vi "230209_Trafficlight_Sync.vi"() -> ()   [LabVIEW 2022 SP3]
panel:
  in  "Standby Off 2":bool
  out "Ampel 2":cluster{"Red":bool, "Orange":bool, "Green":bool}
  out "Ampel":cluster{"Red":bool, "Orange":bool, "Green":bool}
  in  "Ampelzustände Ampel 1":T1(ring)
  in  "Standby Off":bool
  in  "Stop":bool
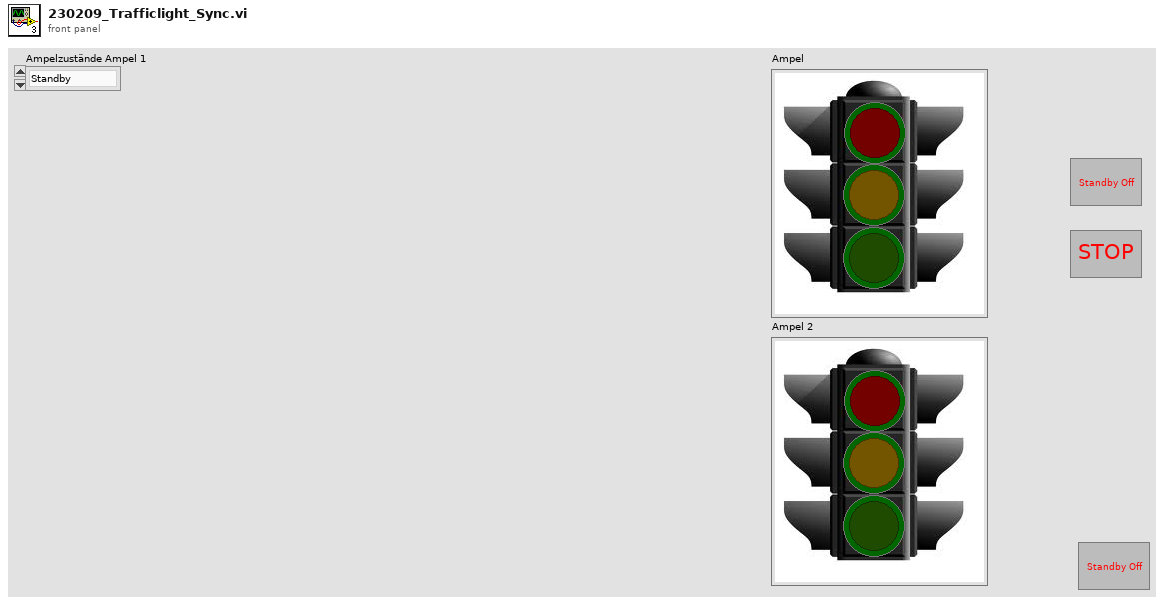
[diagram p1: front panel]
types:
  T1 = enum16{"Standby", "Red", "RedOrange", "Orange", "Green", "GreenBlinking"}
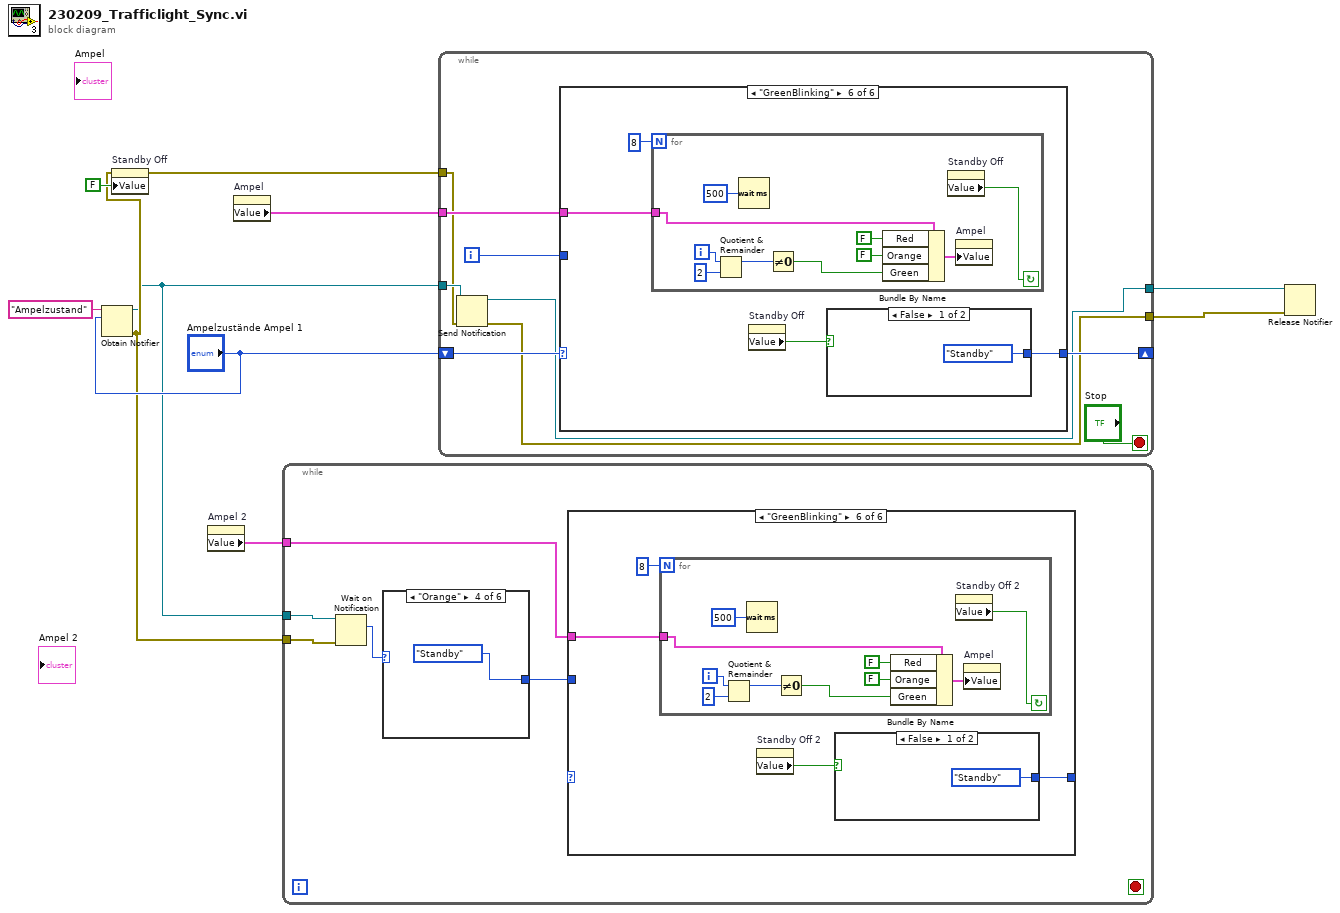
[diagram p0: block diagram]
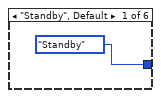
[diagram p2: hidden frame]
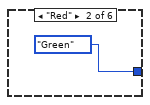
[diagram p3: hidden frame]
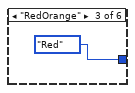
[diagram p4: hidden frame]
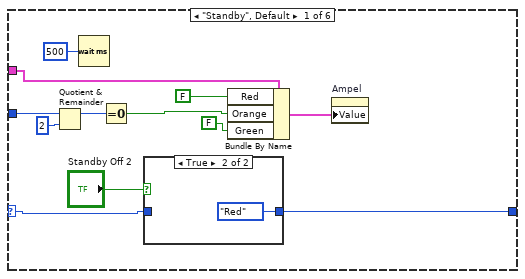
[diagram p7: hidden frame]
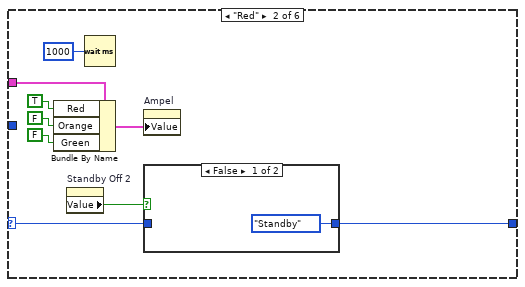
[diagram p9: hidden frame]
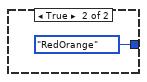
[diagram p10: hidden frame]
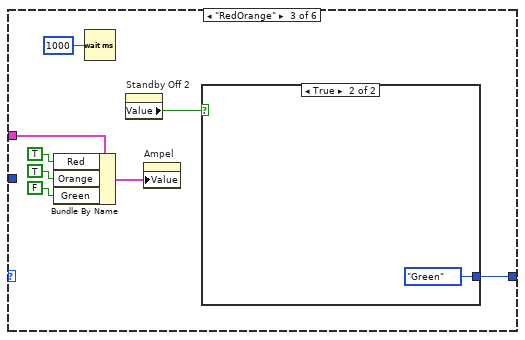
[diagram p11: hidden frame]
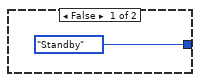
[diagram p12: hidden frame]
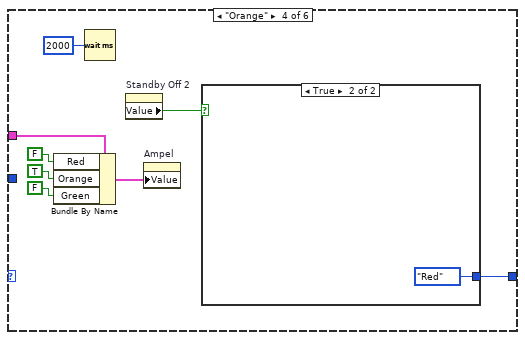
[diagram p13: hidden frame]
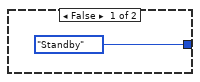
[diagram p14: hidden frame]
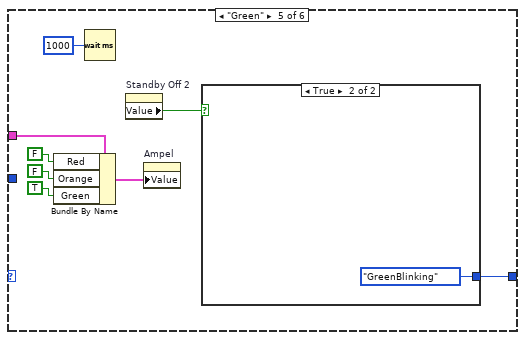
[diagram p15: hidden frame]
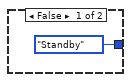
[diagram p16: hidden frame]
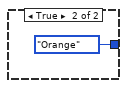
[diagram p17: hidden frame]
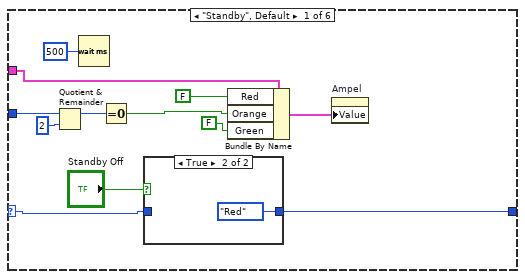
[diagram p18: hidden frame]
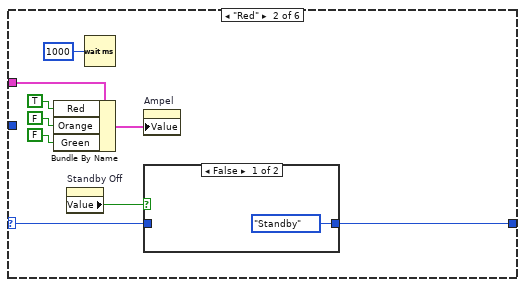
[diagram p20: hidden frame]
diagram:
  n1 = Obtain Notifier(name (unnamed)="Ampelzustand", notification data type="Ampelzustände Ampel 1") -> (notifier out=w2:refnum<notifier>, error out=w3:errorcluster)  [unwired: 2 in, 1 out]
  n2 = property on="Standby Off" class="Bool (strict)"(error in=w3, "Value"=FALSE ("Standby Off")) -> (error out=w8:errorcluster)  [unwired: 1 in, 1 out]
  n3 = property on="Ampel 2" class="Clust (strict)"() -> ("Value"=w1:cluster{"Red":bool, "Orange":bool, "Green":bool})  [unwired: 2 in, 2 out]
  n4 = property on="Ampel" class="Clust (strict)"() -> ("Value"=w10:cluster{"Red":bool, "Orange":bool, "Green":bool})  [unwired: 2 in, 2 out]
  n5 = while {
    tunnel: w3 -> [w15]
    tunnel: w2 -> [w14]
    tunnel: w1 -> [w13]
    stop <- _ stop-if-true
    n6 = Wait on Notification(notifier=w14, error in (no error)=w15) -> (notification=w12:T1)  [unwired: 2 in, 3 out]
    n7 = case shown="\"Orange\"" w12 {
      tunnel: [T1."Standby" ("Enum") T1."Green" ("Enum") T1."Red" ("Enum") T1."Standby" ("Enum") _ _] -> w11
      frame "Standby", Default {
      }
      frame "Red" {
      }
      frame "RedOrange" {
      }
      frame "Orange" {
      }
      frame "Green" {
      }
      frame "GreenBlinking" {
      }
    }
    n8 = case shown="\"GreenBlinking\"" {
      selector: _ -> [w24 w35 _ _ _ _]
      tunnel: w13 -> [w31 w41 w46 w56 w65 w77]
      tunnel: w11 -> [w25 _ _ _ _ _]
      tunnel: [w22 w34 w47 w55 w66 w76] -> _
      frame "Standby", Default {
        n9 = Quotient & Remainder(x=w25, y=2) -> (x-y*floor(x/y)=w27:i32)  [unwired: 1 out]
        n10 = Wait (ms)(milliseconds to wait=u32 500) -> ()  [unwired: 1 out]
        n11 = Equal To 0?(x=w27) -> (x = 0?=w26:bool)
        n12 = case shown="True" "Standby Off 2" {
          tunnel: w24 -> [w32 _]
          tunnel: [w32 T1."Red" ("Enum")] -> w22
          frame False {
          }
          frame True {
          }
        }
        n13 = Bundle By Name(cluster=w31, "Red"=FALSE, "Orange"=w26, "Green"=FALSE) -> (w30:cluster{"Red":bool, "Orange":bool, "Green":bool})
        n14 = property on="Ampel" class="Clust (strict)"("Value"=w30) -> ()  [unwired: 2 in, 2 out]
      }
      frame "Red" {
        n15 = Bundle By Name(cluster=w41, "Red"=TRUE, "Orange"=FALSE, "Green"=FALSE) -> (w42:cluster{"Red":bool, "Orange":bool, "Green":bool})
        n16 = property on="Standby Off 2" class="Bool (strict)"() -> ("Value"=w36:bool)  [unwired: 2 in, 2 out]
        n17 = Wait (ms)(milliseconds to wait=u32 1000) -> ()  [unwired: 1 out]
        n18 = property on="Ampel" class="Clust (strict)"("Value"=w42) -> ()  [unwired: 2 in, 2 out]
        n19 = case shown="False" w36 {
          tunnel: [T1."Standby" ("Enum") T1."RedOrange" ("Enum")] -> w34
          tunnel: w35 -> [_ _]
          frame False {
          }
          frame True {
          }
        }
      }
      frame "RedOrange" {
        n20 = Bundle By Name(cluster=w46, "Red"=TRUE, "Orange"=TRUE, "Green"=FALSE) -> (w45:cluster{"Red":bool, "Orange":bool, "Green":bool})
        n21 = Wait (ms)(milliseconds to wait=u32 1000) -> ()  [unwired: 1 out]
        n22 = property on="Standby Off 2" class="Bool (strict)"() -> ("Value"=w48:bool)  [unwired: 2 in, 2 out]
        n23 = property on="Ampel" class="Clust (strict)"("Value"=w45) -> ()  [unwired: 2 in, 2 out]
        n24 = case shown="True" w48 {
          tunnel: [T1."Standby" ("Enum") T1."Green" ("Enum")] -> w47
          frame False {
          }
          frame True {
          }
        }
      }
      frame "Orange" {
        n25 = Bundle By Name(cluster=w56, "Red"=FALSE, "Orange"=TRUE, "Green"=FALSE) -> (w61:cluster{"Red":bool, "Orange":bool, "Green":bool})
        n26 = Wait (ms)(milliseconds to wait=u32 2000) -> ()  [unwired: 1 out]
        n27 = property on="Standby Off 2" class="Bool (strict)"() -> ("Value"=w62:bool)  [unwired: 2 in, 2 out]
        n28 = property on="Ampel" class="Clust (strict)"("Value"=w61) -> ()  [unwired: 2 in, 2 out]
        n29 = case shown="True" w62 {
          tunnel: [T1."Standby" ("Enum") T1."Red" ("Enum")] -> w55
          frame False {
          }
          frame True {
          }
        }
      }
      frame "Green" {
        n30 = Bundle By Name(cluster=w65, "Red"=FALSE, "Orange"=FALSE, "Green"=TRUE) -> (w71:cluster{"Red":bool, "Orange":bool, "Green":bool})
        n31 = Wait (ms)(milliseconds to wait=u32 1000) -> ()  [unwired: 1 out]
        n32 = property on="Standby Off 2" class="Bool (strict)"() -> ("Value"=w72:bool)  [unwired: 2 in, 2 out]
        n33 = property on="Ampel" class="Clust (strict)"("Value"=w71) -> ()  [unwired: 2 in, 2 out]
        n34 = case shown="True" w72 {
          tunnel: [T1."Standby" ("Enum") T1."GreenBlinking" ("Enum")] -> w66
          frame False {
          }
          frame True {
          }
        }
      }
      frame "GreenBlinking" {
        n35 = for {
          N: 8 -> [_]
          tunnel: w77 -> [w84]
          i -> [w82]
          stop <- w79 continue-if-true
          n36 = Quotient & Remainder(x=w82, y=2) -> (x-y*floor(x/y)=w81:i32)  [unwired: 1 out]
          n37 = Wait (ms)(milliseconds to wait=u32 500) -> ()  [unwired: 1 out]
          n38 = Not Equal To 0?(x=w81) -> (x != 0?=w80:bool)
          n39 = Bundle By Name(cluster=w84, "Red"=FALSE, "Orange"=FALSE, "Green"=w80) -> (w83:cluster{"Red":bool, "Orange":bool, "Green":bool})
          n40 = property on="Standby Off 2" class="Bool (strict)"() -> ("Value"=w79:bool)  [unwired: 2 in, 2 out]
          n41 = property on="Ampel" class="Clust (strict)"("Value"=w83) -> ()  [unwired: 2 in, 2 out]
        }
        n42 = property on="Standby Off 2" class="Bool (strict)"() -> ("Value"=w78:bool)  [unwired: 2 in, 2 out]
        n43 = case shown="False" w78 {
          tunnel: [T1."Standby" ("Enum") T1."Orange" ("Enum")] -> w76
          frame False {
          }
          frame True {
          }
        }
      }
    }
  }
  n44 = while {
    shift-right: [w95] -> _
    shift-left: "Ampelzustände Ampel 1" -> [w97]
    tunnel: w10 -> [w98]
    tunnel: w8 -> [w92]
    tunnel: w2 -> [w94]
    tunnel: [w93] -> w5
    tunnel: [w91] -> w4
    i -> [w96]
    stop <- "Stop" stop-if-true
    n45 = Send Notification(notifier=w94, error in (no error)=w92) -> (notifier out=w93:refnum<notifier>, error out=w91:errorcluster)  [unwired: 1 in]
    n46 = case shown="\"GreenBlinking\"" w97 {
      selector: w97 -> [w104 w115 _ _ _ _]
      tunnel: w98 -> [w111 w121 w126 w136 w145 w157]
      tunnel: w96 -> [w105 _ _ _ _ _]
      tunnel: [w102 w114 w127 w135 w146 w156] -> w95
      frame "Standby", Default {
        n47 = Quotient & Remainder(x=w105, y=2) -> (x-y*floor(x/y)=w107:i32)  [unwired: 1 out]
        n48 = Wait (ms)(milliseconds to wait=u32 500) -> ()  [unwired: 1 out]
        n49 = Equal To 0?(x=w107) -> (x = 0?=w106:bool)
        n50 = case shown="True" "Standby Off" {
          tunnel: w104 -> [w112 _]
          tunnel: [w112 T1."Red" ("Enum")] -> w102
          frame False {
          }
          frame True {
          }
        }
        n51 = Bundle By Name(cluster=w111, "Red"=FALSE, "Orange"=w106, "Green"=FALSE) -> (w110:cluster{"Red":bool, "Orange":bool, "Green":bool})
        n52 = property on="Ampel" class="Clust (strict)"("Value"=w110) -> ()  [unwired: 2 in, 2 out]
      }
      frame "Red" {
        n53 = Bundle By Name(cluster=w121, "Red"=TRUE, "Orange"=FALSE, "Green"=FALSE) -> (w122:cluster{"Red":bool, "Orange":bool, "Green":bool})
        n54 = property on="Standby Off" class="Bool (strict)"() -> ("Value"=w116:bool)  [unwired: 2 in, 2 out]
        n55 = Wait (ms)(milliseconds to wait=u32 1000) -> ()  [unwired: 1 out]
        n56 = property on="Ampel" class="Clust (strict)"("Value"=w122) -> ()  [unwired: 2 in, 2 out]
        n57 = case shown="False" w116 {
          tunnel: [T1."Standby" ("Enum") T1."RedOrange" ("Enum")] -> w114
          tunnel: w115 -> [_ _]
          frame False {
          }
          frame True {
          }
        }
      }
      frame "RedOrange" {
        n58 = Bundle By Name(cluster=w126, "Red"=TRUE, "Orange"=TRUE, "Green"=FALSE) -> (w125:cluster{"Red":bool, "Orange":bool, "Green":bool})
        n59 = Wait (ms)(milliseconds to wait=u32 1000) -> ()  [unwired: 1 out]
        n60 = property on="Standby Off" class="Bool (strict)"() -> ("Value"=w128:bool)  [unwired: 2 in, 2 out]
        n61 = property on="Ampel" class="Clust (strict)"("Value"=w125) -> ()  [unwired: 2 in, 2 out]
        n62 = case shown="True" w128 {
          tunnel: [T1."Standby" ("Enum") T1."Green" ("Enum")] -> w127
          frame False {
          }
          frame True {
          }
        }
      }
      frame "Orange" {
        n63 = Bundle By Name(cluster=w136, "Red"=FALSE, "Orange"=TRUE, "Green"=FALSE) -> (w141:cluster{"Red":bool, "Orange":bool, "Green":bool})
        n64 = Wait (ms)(milliseconds to wait=u32 2000) -> ()  [unwired: 1 out]
        n65 = property on="Standby Off" class="Bool (strict)"() -> ("Value"=w142:bool)  [unwired: 2 in, 2 out]
        n66 = property on="Ampel" class="Clust (strict)"("Value"=w141) -> ()  [unwired: 2 in, 2 out]
        n67 = case shown="True" w142 {
          tunnel: [T1."Standby" ("Enum") T1."Red" ("Enum")] -> w135
          frame False {
          }
          frame True {
          }
        }
      }
      frame "Green" {
        n68 = Bundle By Name(cluster=w145, "Red"=FALSE, "Orange"=FALSE, "Green"=TRUE) -> (w151:cluster{"Red":bool, "Orange":bool, "Green":bool})
        n69 = Wait (ms)(milliseconds to wait=u32 1000) -> ()  [unwired: 1 out]
        n70 = property on="Standby Off" class="Bool (strict)"() -> ("Value"=w152:bool)  [unwired: 2 in, 2 out]
        n71 = property on="Ampel" class="Clust (strict)"("Value"=w151) -> ()  [unwired: 2 in, 2 out]
        n72 = case shown="True" w152 {
          tunnel: [T1."Standby" ("Enum") T1."GreenBlinking" ("Enum")] -> w146
          frame False {
          }
          frame True {
          }
        }
      }
      frame "GreenBlinking" {
        n73 = for {
          N: 8 -> [_]
          tunnel: w157 -> [w164]
          i -> [w162]
          stop <- w159 continue-if-true
          n74 = Quotient & Remainder(x=w162, y=2) -> (x-y*floor(x/y)=w161:i32)  [unwired: 1 out]
          n75 = Wait (ms)(milliseconds to wait=u32 500) -> ()  [unwired: 1 out]
          n76 = Not Equal To 0?(x=w161) -> (x != 0?=w160:bool)
          n77 = Bundle By Name(cluster=w164, "Red"=FALSE, "Orange"=FALSE, "Green"=w160) -> (w163:cluster{"Red":bool, "Orange":bool, "Green":bool})
          n78 = property on="Standby Off" class="Bool (strict)"() -> ("Value"=w159:bool)  [unwired: 2 in, 2 out]
          n79 = property on="Ampel" class="Clust (strict)"("Value"=w163) -> ()  [unwired: 2 in, 2 out]
        }
        n80 = property on="Standby Off" class="Bool (strict)"() -> ("Value"=w158:bool)  [unwired: 2 in, 2 out]
        n81 = case shown="False" w158 {
          tunnel: [T1."Standby" ("Enum") T1."Orange" ("Enum")] -> w156
          frame False {
          }
          frame True {
          }
        }
      }
    }
  }
  n82 = Release Notifier(notifier=w5, error in (no error)=w4) -> ()  [unwired: 1 in, 3 out]
